vi "constructTopicControl.vi"(8 "error in (no error)":errorcluster, 10 "libraryInfo":T1, 11 "Topic in":refnum<class "Topic.lvclass">) -> (0 "error out":errorcluster, 3 "Topic out":refnum<class "Topic.lvclass">)   [LabVIEW 2016, in "Topic.lvclass"]
uses:
  Topic.lvclass
  Typedefs/LibraryInfo.ctl
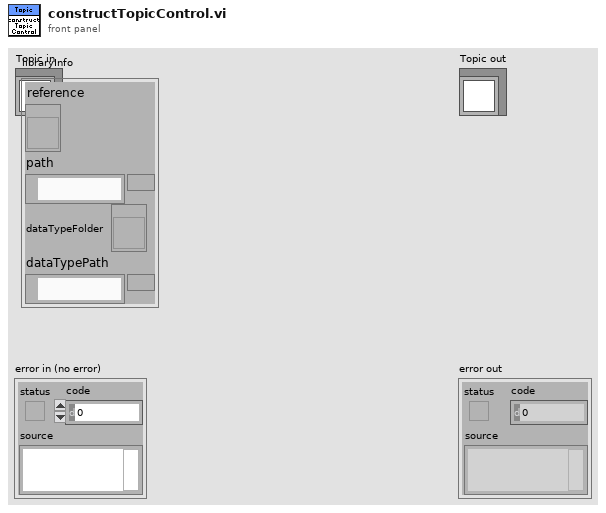
[diagram p1: front panel]
types:
  T1 = typedef "LibraryInfo.ctl" = cluster{"reference":refnum<vi>, "path":path, "dataTypeFolder":refnum<vi>, "dataTypePath":path}
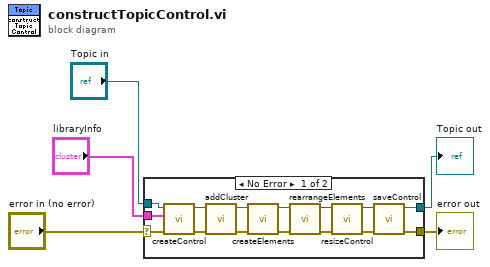
[diagram p0: block diagram]
diagram:
  n1 = case shown="No Error" "error in (no error)" {
    selector: "error in (no error)" -> [w19 w22]
    tunnel: [w14 w22] -> w4
    tunnel: [w15 w21] -> w2
    tunnel: "Topic in" -> [w16 w21]
    tunnel: "libraryInfo" -> [w20 _]
    frame No Error {
      n2 = call "createControl.vi"("error in (no error)"=w19, "LibraryInfo"=w20, "Topic in"=w16) -> ("error out"=w17:errorcluster, "Topic out"=w18:refnum<class "Topic.lvclass">)  [unwired: 7 in]
      n3 = call "addCluster.vi"("error in (no error)"=w17, "Topic in"=w18) -> ("error out"=w12:errorcluster, "Topic out"=w13:refnum<class "Topic.lvclass">)  [unwired: 8 in]
      n4 = call "createElements.vi"("error in (no error)"=w12, "Topic in"=w13) -> ("error out"=w10:errorcluster, "Topic out"=w11:refnum<class "Topic.lvclass">)  [unwired: 8 in]
      n5 = call "rearrangeElements.vi"("error in (no error)"=w10, "Topic in"=w11) -> ("error out"=w8:errorcluster, "Topic out"=w9:refnum<class "Topic.lvclass">)  [unwired: 8 in]
      n6 = call "resizeControl.vi"("error in (no error)"=w8, "Topic in"=w9) -> ("error out"=w6:errorcluster, "Topic out"=w7:refnum<class "Topic.lvclass">)  [unwired: 8 in]
      n7 = call "saveControl.vi"("error in (no error)"=w6, "Topic in"=w7) -> ("error out"=w14:errorcluster, "Topic out"=w15:refnum<class "Topic.lvclass">)  [unwired: 8 in]
    }
    frame Error {
    }
  }
  "error out" <- w4
  "Topic out" <- w2
